vi "Compare System Configuration.vi"(8 "error in (no error)":errorcluster, 10 "New System Configuration":T2, 11 "System Configuration":T2) -> (0 "error out":errorcluster, 1 "Changed?":bool, 2 "Subsystems Deleted":T1[](array[typedef]), 3 "Subsystems Added":T1[](array[typedef]))   [LabVIEW 2024]
doc: "Compares the new system configuration with the previous system configuration and judges whether the configuration has changed."
uses:
  Controls/Server/System Configuration.ctl
  Controls/Server/Subsystem Configuration.ctl
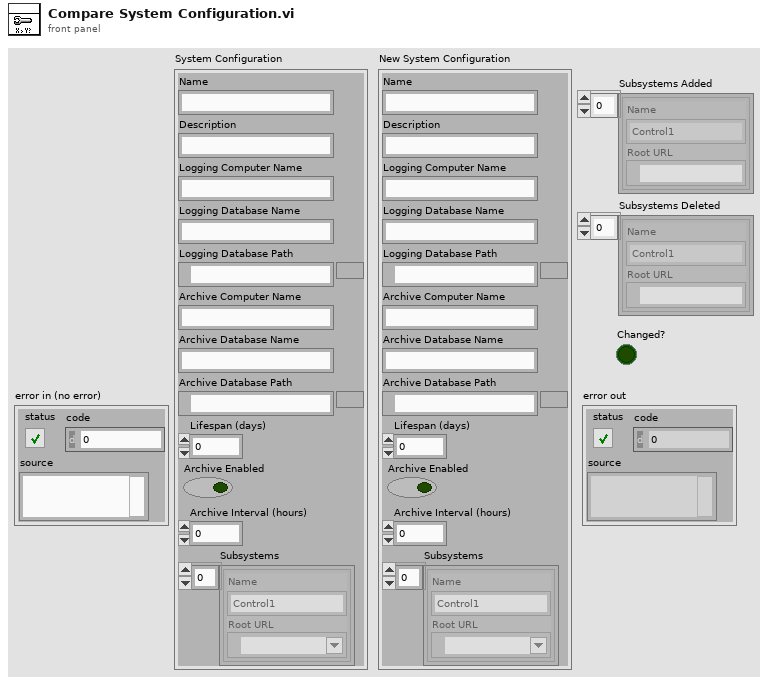
[diagram p1: front panel]
types:
  T1 = typedef "Subsystem Configuration.ctl" = cluster{"Name":string, "Root URL":refnum<k21>}
  T2 = typedef "System Configuration.ctl" = cluster{"Name":string, "Description":string, "Logging Computer Name":string, "Logging Database Name":string, "Logging Database Path":path, "Archive Computer Name":string, "Archive Database Name":string, "Archive Database Path":path, "Lifespan (days)":u32, "Archive Enabled":bool, "Archive Interval (hours)":u32, "Subsystems":T1[]}
  T3 = cluster{"Name":string, "Description":string, "Logging Computer Name":string, "Logging Database Name":string, "Logging Database Path":path, "Lifespan (days)":u32, "Archive Enabled":bool, "Archive Computer Name":string, "Archive Database Name":string, "Archive Database Path":path, "Archive Interval (hours)":u32}
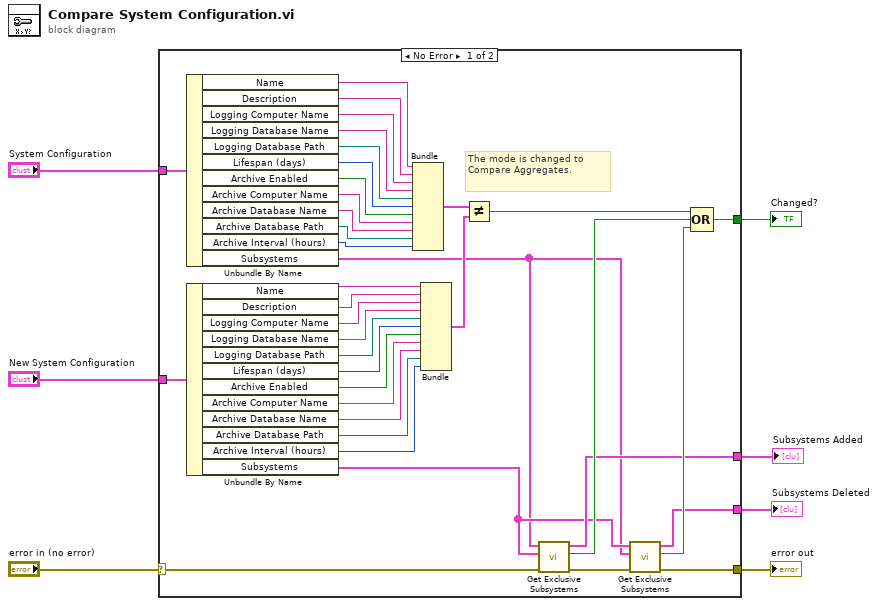
[diagram p0: block diagram]
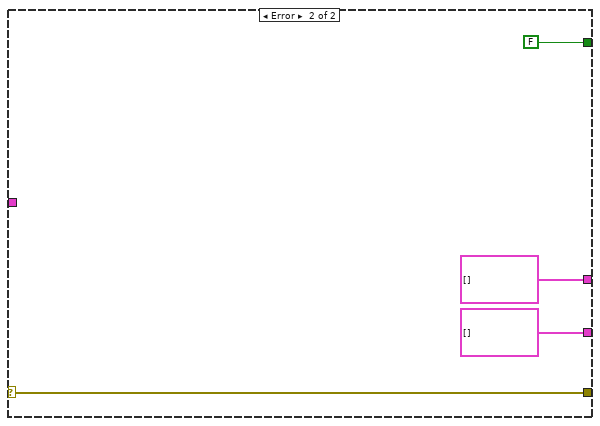
[diagram p2: hidden frame]
diagram:
  n1 = case shown="No Error" "error in (no error)" {
    selector: "error in (no error)" -> [w42 w48]
    tunnel: [w40 w48] -> w7
    tunnel: "System Configuration" -> [w44 _]
    tunnel: "New System Configuration" -> [w43 _]
    tunnel: [w15 FALSE] -> w4
    tunnel: [w12 T1[] [] ("Subsystems to be added")] -> w3
    tunnel: [w11 T1[] [] ("Subsystems to be deleted")] -> w2
    frame No Error {
      # "The mode is changed to Compare Aggregates."
      n2 = Unbundle By Name(w44) -> ("Name"=w39:string, "Description"=w38:string, "Logging Computer Name"=w37:string, "Logging Database Name"=w36:string, "Logging Database Path"=w35:path, "Lifespan (days)"=w34:u32, "Archive Enabled"=w33:bool, "Archive Computer Name"=w32:string, "Archive Database Name"=w31:string, "Archive Database Path"=w30:path, "Archive Interval (hours)"=w29:u32, "Subsystems"=w9:T1[])
      n3 = Unbundle By Name(w43) -> ("Name"=w28:string, "Description"=w27:string, "Logging Computer Name"=w26:string, "Logging Database Name"=w25:string, "Logging Database Path"=w24:path, "Lifespan (days)"=w23:u32, "Archive Enabled"=w22:bool, "Archive Computer Name"=w21:string, "Archive Database Name"=w20:string, "Archive Database Path"=w19:path, "Archive Interval (hours)"=w18:u32, "Subsystems"=w10:T1[])
      n4 = Bundle("Name"=w39, "Description"=w38, "Logging Computer Name"=w37, "Logging Database Name"=w36, "Logging Database Path"=w35, "Lifespan (days)"=w34, "Archive Enabled"=w33, "Archive Computer Name"=w32, "Archive Database Name"=w31, "Archive Database Path"=w30, "Archive Interval (hours)"=w29) -> (w16:T3)  [unwired: 1 in]
      n5 = Bundle("Name"=w28, "Description"=w27, "Logging Computer Name"=w26, "Logging Database Name"=w25, "Logging Database Path"=w24, "Lifespan (days)"=w23, "Archive Enabled"=w22, "Archive Computer Name"=w21, "Archive Database Name"=w20, "Archive Database Path"=w19, "Archive Interval (hours)"=w18) -> (w17:T3)  [unwired: 1 in]
      n6 = Not Equal?(x=w16, y=w17) -> (x != y?=w8:bool)
      n7 = call "Get Exclusive Subsystems.vi"("error in (no error)"=w42, "Subsystem Array B"=w10, "Subsystem Array A"=w9) -> ("error out"=w41:errorcluster, "Exist?"=w14:bool, "Exclusive Subsystems"=w12:T1[])  [unwired: 6 in]
      n8 = call "Get Exclusive Subsystems.vi"("error in (no error)"=w41, "Subsystem Array B"=w9, "Subsystem Array A"=w10) -> ("error out"=w40:errorcluster, "Exist?"=w13:bool, "Exclusive Subsystems"=w11:T1[])  [unwired: 6 in]
      n9 = Compound Arithmetic op=OR(w8, w14, w13) -> (w15:bool)
    }
    frame Error {
    }
  }
  "error out" <- w7
  "Changed?" <- w4
  "Subsystems Deleted" <- w2
  "Subsystems Added" <- w3
